vi "Generate Serial String.vi"(0 "Dynamixel Motor VISA in":refnum<class "Dynamixel Motor VISA.lvclass">, 5 "Motor ID":u8, 7 "Command":u8, 9 "Address":u8, 11 "error in (no error)":errorcluster, 12 "Parameters":string) -> (4 "Dynamixel Motor VISA out":refnum<class "Dynamixel Motor VISA.lvclass">, 6 "Command to Serial":string, 15 "error out":errorcluster)   [LabVIEW 2016, in "Dynamixel Motor VISA.lvclass"]
doc: "Generates a valid serial string that can be sent to the motor(s). This is a Low-Level VI that is used by other VIs."
uses:
  <instrlib>/Dynamixel Motor/HAIOL/VISA/Dynamixel Motor VISA.lvclass
  <instrlib>/Dynamixel Motor/Dynamixel Motor.lvlib
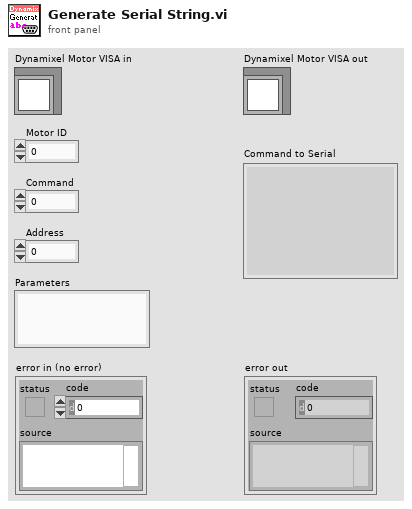
[diagram p1: front panel]
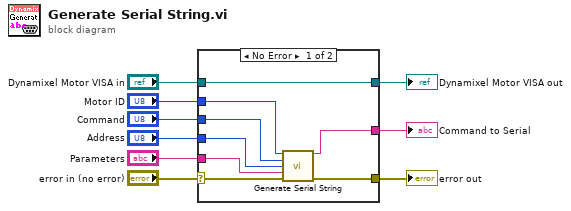
[diagram p0: block diagram]
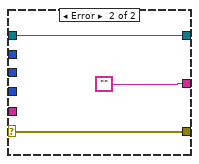
[diagram p2: hidden frame]
diagram:
  n1 = case shown="No Error" "error in (no error)" {
    selector: "error in (no error)" -> [w17 w19]
    tunnel: "Dynamixel Motor VISA in" -> [w10 w18]
    tunnel: "Motor ID" -> [w16 _]
    tunnel: "Command" -> [w15 _]
    tunnel: "Address" -> [w14 _]
    tunnel: "Parameters" -> [w13 _]
    tunnel: [w12 w19] -> w3
    tunnel: [w11 ""] -> w2
    tunnel: [w10 w18] -> w1
    frame No Error {
      n2 = call <instrlib>:"Generate Serial String.vi"("Motor ID"=w16, "Command"=w15, "Address"=w14, "Parameters"=w13, "Error in (no error)"=w17) -> ("Command to Serial"=w11:string, "error out"=w12:errorcluster)  [unwired: 9 in]
    }
    frame Error {
    }
  }
  "error out" <- w3
  "Dynamixel Motor VISA out" <- w1
  "Command to Serial" <- w2
